vi "串口通讯模块.vi"(1 "发送区":string, 4 "校检":u16, 5 "数据位":u16, 6 "波特率":u16, 7 "VISA resource name":refnum<visa-resource-name>) -> (0 "接收区":string)   [LabVIEW 2015, in "PLC.lvlib"]
uses:
  <vilib>/Instr/_visa.llb/VISA Configure Serial Port (Instr).vi
  PLC.lvlib
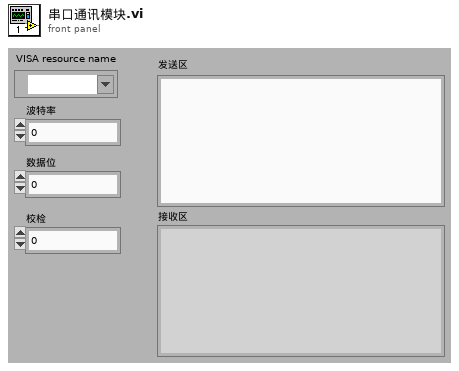
[diagram p1: front panel]
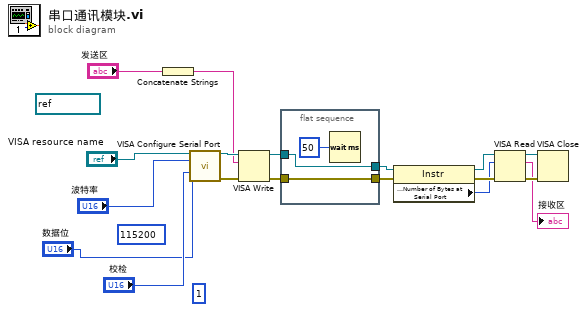
[diagram p0: block diagram]
diagram:
  (unwired) 1
  (unwired) 115200
  (unwired) refnum<visa-resource-name> "COM1" ("VISA resource name")
  n1 = Concatenate Strings("发送区") -> (w6:string)
  n2 = call-poly "VISA Configure Serial Port"("VISA resource name"="VISA resource name", "baud rate (9600)"="波特率", "data bits (8)"="数据位", "parity (0:none)"="校检") -> ("VISA resource name out"=w8:refnum<visa-resource-name>, "error out"=w7:errorcluster)  [unwired: 2 in, 8 out]
  n3 = VISA Write(VISA resource name=w8, write buffer=w6, error in (no error)=w7) -> (VISA resource name out=w17:refnum<visa-resource-name>, error out=w15:errorcluster)  [unwired: 1 out]
  n4 = flat-sequence {
    tunnel: [w20] -> w18
    tunnel: w17 -> [w20]
    tunnel: [w19] -> w16
    tunnel: w15 -> [w19]
    frame #0 {
      n5 = Wait (ms)(milliseconds to wait=50) -> ()  [unwired: 1 out]
    }
  }
  n6 = property class="Instr"(reference=w18, error in=w16) -> (reference out=w12:refnum<visa-resource-name>, error out=w14:errorcluster, "Serial Settings:Number of Bytes at Serial Port"=w11:u32)
  n7 = VISA Read(VISA resource name=w12, byte count=w11, error in (no error)=w14) -> (VISA resource name out=w9:refnum<visa-resource-name>, read buffer=→"接收区":string, error out=w13:errorcluster)  [unwired: 1 out]
  n8 = VISA Close(VISA resource name=w9, error in (no error)=w13) -> ()  [unwired: 1 out]
